vi "624WPI_DashboardReceive DS Packet.vi"(0 "Recv Socket":refnum<k16>, 5 "Log User Data":bool) -> (2 "New Dashboard Data":bool, 3 "Battery":sgl, 4 "Error Strings":string, 6 "Driver Station":T1, 8 "Robot IP Address":string="10.0.0.2", 10 "Status":T3, 12 "Camera IP Address":string="10.0.0.2", 13 "Low Priority User Data":string, 14 "High Priority User Data":string, 15 "Error":T2)   [LabVIEW 2013]
uses:
  <vilib>/Rock Robotics/WPI/Dashboard/WPI_DashboardDStoPCPacketTypeDef.ctl
  <vilib>/Rock Robotics/WPI/Dashboard/WPI_DashboardLogging Global.vi
panel:
  out "Team ID":u16
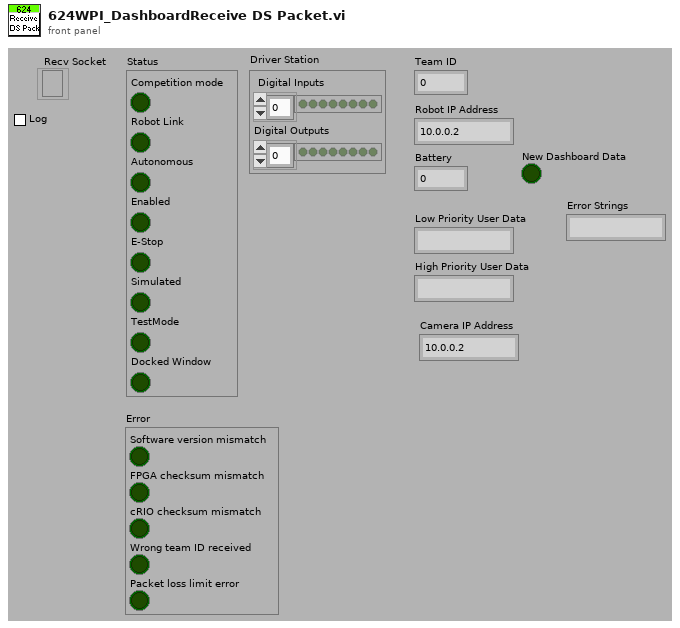
[diagram p1: front panel]
types:
  T1 = cluster{"Digital Inputs":bool[], "Digital Outputs":bool[]}
  T2 = cluster{"Software version mismatch":bool, "FPGA checksum mismatch":bool, "cRIO checksum mismatch":bool, "Wrong team ID received":bool, "Packet loss limit error":bool}
  T3 = cluster{"Competition mode":bool, "Robot Link":bool, "Autonomous":bool, "Enabled":bool, "E-Stop":bool, "Simulated":bool, "TestMode":bool, "Docked Window":bool}
  T4 = typedef "WPI_DashboardDStoPCPacketTypeDef.ctl" = cluster{"Packet Index":u16, "Digital Inputs":u8, "Digital Out":u8, "Battery":u16, "Status":u8, "Error":u8, "Team ID":u16, "VersionMonth1":u8, "VersionMonth2":u8, "VersionDay1":u8, "VersionDay2":u8, "VersionYear1":u8, "VersionYear2":u8, "Revision1":u8, "Revision2":u8, "Robot IP":u32, "UnusedBuffer 2":u8, "ExtraModeFlags":u8, "Reply Packet #":u16}
  T5 = cluster{u16, "Error":cluster{"Software version mismatch":bool, "FPGA checksum mismatch":bool, "cRIO checksum mismatch":bool, "Wrong team ID received":bool, "Packet loss limit error":bool}, "Status":cluster{"Competition mode":bool, "Robot Link":bool, "Autonomous":bool, "Enabled":bool, "E-Stop":bool, "Simulated":bool, "TestMode":bool, "Docked Window":bool}, "Simulator":bool, cluster{"DS Dig Inputs":bool[], "DS Dig Outputs":bool[]}, "Battery":sgl, "name":string}
  T6 = cluster{"DS Dig Inputs":bool[], "DS Dig Outputs":bool[]}
  T7 = typedef "Vector4.ctl" = cluster{"x":sgl, "y":sgl, "z":sgl, "w":sgl}
  T8 = typedef "SkeletonTrackState.ctl" = enum32{"NotTracked", "PositionOnly", "Tracked"}
  T9 = typedef "WPI_JoystickDeviceDataRaw.ctl" = cluster{"axis 1":i8, "axis 2":i8, "axis 3":i8, "axis 4":i8, "axis 5":i8, "axis 6":i8, "Buttons":u16}
  T10 = cluster{"size":u8, "tag":u8, "Version":cluster{"unsigned byte array[0]":u8, "unsigned byte array[1]":u8, "unsigned byte array[2]":u8, "unsigned byte array[3]":u8, "unsigned byte array[4]":u8, "unsigned byte array[5]":u8, "unsigned byte array[6]":u8, "unsigned byte array[7]":u8, "unsigned byte array[8]":u8, "unsigned byte array[9]":u8, "unsigned byte array[10]":u8}, "numPlayers":i8, "flags":u32, "floorClipPlane":T7, "Gravity Normal":cluster{"x":sgl, "y":sgl, "z":sgl}, "size":u8, "tag":u8, "Extra Data":cluster{"TrackingState":cluster{"TrackingState[0]":u8, "TrackingState[1]":u8, "TrackingState[2]":u8, "TrackingState[3]":u8, "TrackingState[4]":u8, "TrackingState[5]":u8, "TrackingState[6]":u8, "TrackingState[7]":u8, "TrackingState[8]":u8, "TrackingState[9]":u8, "TrackingState[10]":u8, "TrackingState[11]":u8, "TrackingState[12]":u8, "TrackingState[13]":u8, "TrackingState[14]":u8, "TrackingState[15]":u8, "TrackingState[16]":u8, "TrackingState[17]":u8, "TrackingState[18]":u8, "TrackingState[19]":u8}, "Position":cluster{"x":sgl, "y":sgl, "z":sgl}, "Quality":u32, "TrackState":T8}, "size":u8, "tag":u8, "Vertices":cluster{"Vertices[0]":cluster{"x":sgl, "y":sgl, "z":sgl}, "Vertices[1]":cluster{"x":sgl, "y":sgl, "z":sgl}, "Vertices[2]":cluster{"x":sgl, "y":sgl, "z":sgl}, "Vertices[3]":cluster{"x":sgl, "y":sgl, "z":sgl}, "Vertices[4]":cluster{"x":sgl, "y":sgl, "z":sgl}, "Vertices[5]":cluster{"x":sgl, "y":sgl, "z":sgl}, "Vertices[6]":cluster{"x":sgl, "y":sgl, "z":sgl}, "Vertices[7]":cluster{"x":sgl, "y":sgl, "z":sgl}, "Vertices[8]":cluster{"x":sgl, "y":sgl, "z":sgl}, "Vertices[9]":cluster{"x":sgl, "y":sgl, "z":sgl}, "Vertices[10]":cluster{"x":sgl, "y":sgl, "z":sgl}, "Vertices[11]":cluster{"x":sgl, "y":sgl, "z":sgl}, "Vertices[12]":cluster{"x":sgl, "y":sgl, "z":sgl}, "Vertices[13]":cluster{"x":sgl, "y":sgl, "z":sgl}, "Vertices[14]":cluster{"x":sgl, "y":sgl, "z":sgl}, "Vertices[15]":cluster{"x":sgl, "y":sgl, "z":sgl}, "Vertices[16]":cluster{"x":sgl, "y":sgl, "z":sgl}, "Vertices[17]":cluster{"x":sgl, "y":sgl, "z":sgl}, "Vertices[18]":cluster{"x":sgl, "y":sgl, "z":sgl}, "Vertices[19]":cluster{"x":sgl, "y":sgl, "z":sgl}}, "size":u8, "tag":u8, "Joystick":T9, "Joystick 2":T9, "size":u8, "tag":u8, "Custom Data":string}[]
  T11 = cluster{"Team ID":u16, "Error":cluster{"Software version mismatch":bool, "FPGA checksum mismatch":bool, "cRIO checksum mismatch":bool, "Wrong team ID received":bool, "Packet loss limit error":bool}, "Status":cluster{"Competition mode":bool, "Robot Link":bool, "Autonomous":bool, "Enabled":bool, "E-Stop":bool, "Simulated":bool, "TestMode":bool, "Docked Window":bool}, "Robot IP":string, "Camera IP":string}
  T12 = cluster{cluster{"Packet #":u8, "High Priority":string, "Error Strings":string, "Low Priority":string}, cluster{"DS Digital In":bool[], "DS Digital Out":bool[]}, "Battery":sgl}
  T13 = cluster{"Packet #":u8, "High Priority":string, "Error Strings":string, "Low Priority":string}
  T14 = cluster{"DS Digital In":bool[], "DS Digital Out":bool[]}
  T15 = cluster{"Team ID":u16, "Error":cluster{"Software version mismatch":bool, "FPGA checksum mismatch":bool, "cRIO checksum mismatch":bool, "Wrong team ID received":bool, "Packet loss limit error":bool}, "Status":cluster{"Competition mode":bool, "Robot Link":bool, "Autonomous":bool, "Enabled":bool, "E-Stop":bool, "Simulated":bool, "TestMode":bool, "Docked Window":bool}, "Camera IP":string, "Camera IP":string}
  T16 = typedef "Protocol Operations.ctl" = enum16{"Unknown", "Keep Alive", "Hello", "Version not supported", "Hello Complete", "Assign", "Update", "No Op"}
  T17 = typedef "Field Data.ctl" = cluster{"Dbl":dbl, "String":string, "Type":T18, "Boolean":bool, "Sequence #":T19}
  T18 = typedef "Field Type.ctl" = enum8{"Invalid", "Bool", "Numeric", "String", "Boolean Array", "Numeric Array", "String Array"}
  T19 = typedef "Sequence.ctl" = u16
  T20 = cluster{"Operation":T16, "Name":string, "Field Value":T17}[]
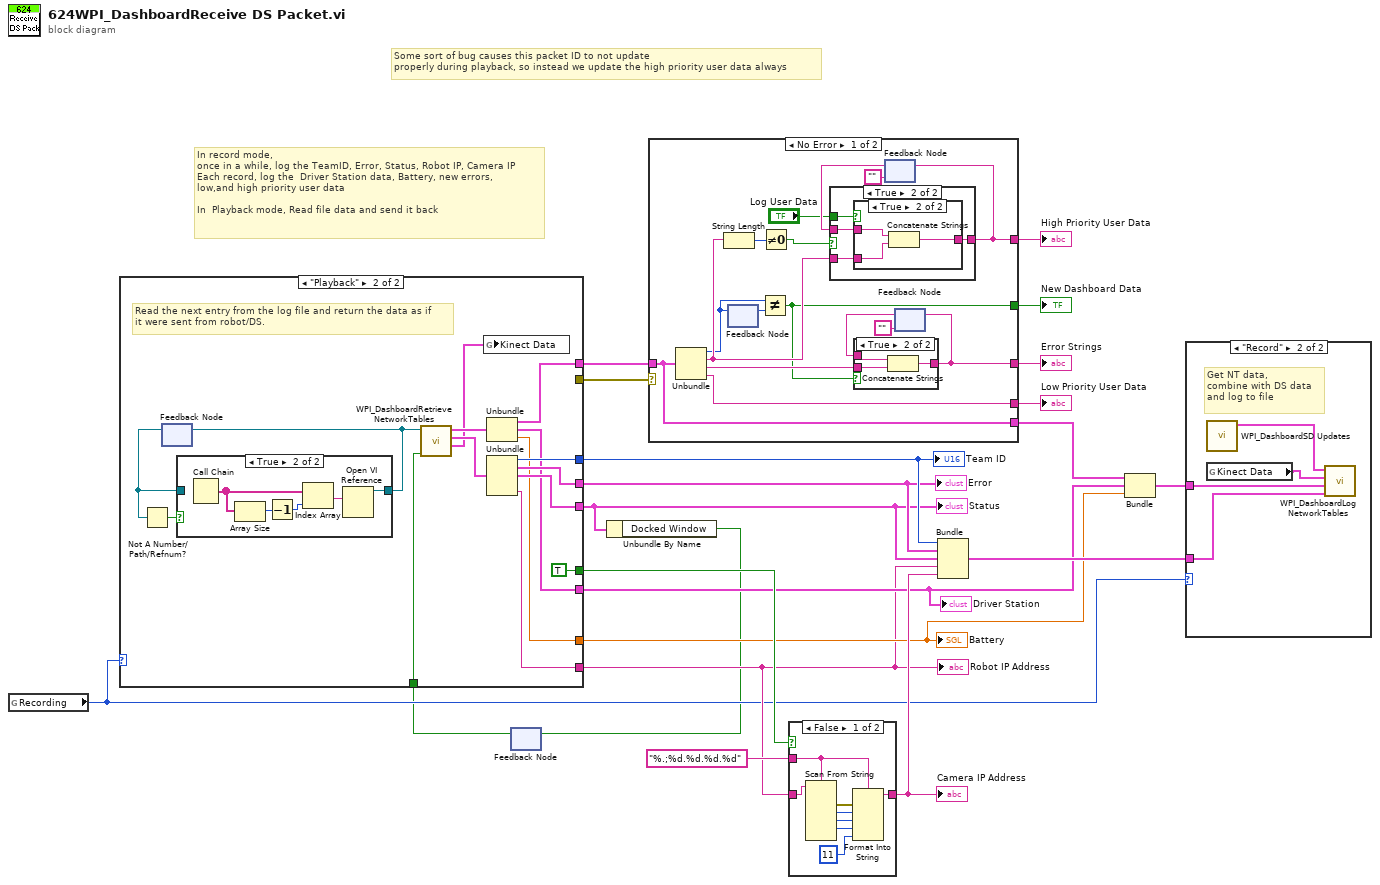
[diagram p0: block diagram]
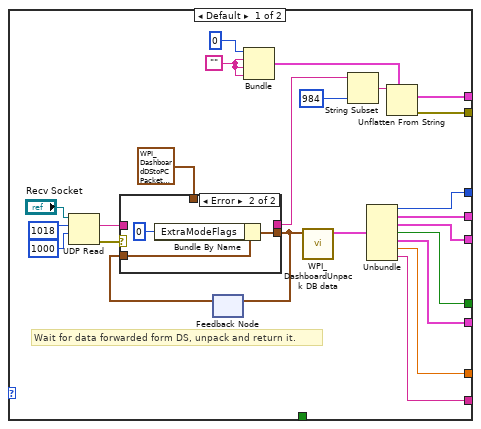
[diagram p3: hidden frame]
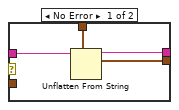
[diagram p4: hidden frame]
diagram:
  # "Some sort of bug causes this packet ID to not update\nproperly during playback, so instead we update the high priority user data always"
  # "In record mode,\nonce in a while, log the TeamID, Error, Status, Robot IP, Camera IP\nEach record, log the  Driver Station data, Battery, new errors,\nlow,and high priority user data\n\nIn  Playback mode, Read file data and send it back"
  n1 = global read "WPI_DashboardLogging Global.vi" "Recording"() -> (w4:enum32{"Stop", "Record", "Playback"})
  n2 = feedback #1() -> (w1:bool)  [unwired: 1 in]
  n3 = case shown="\"Playback\"" w4 {
    tunnel: [w32 _] -> w12
    tunnel: [w31 w66] -> w11
    tunnel: [w29 w64] -> w10
    tunnel: [w28 w63] -> w9
    tunnel: [w27 w62] -> w3
    tunnel: [w26 TRUE] -> w8
    tunnel: [w25 w61] -> w7
    tunnel: [w24 w60] -> w6
    tunnel: [w23 w53] -> w5
    tunnel: w1 -> [_ w55]
    frame Default {
      w39 = ""
      # "Wait for data forwarded form DS, unpack and return it."
      n4 = UDP Read(connection ID="Recv Socket", max size (548)=1018 ("bytes to read"), timeout ms (25000)=1000) -> (data out=w34:string, error out=w33:errorcluster)  [unwired: 1 in, 3 out]
      n5 = feedback #2() -> (w40:T4)  [unwired: 1 in]
      n6 = case shown="Error" w33 {
        tunnel: w34 -> [w49 _]
        tunnel: w40 -> [_ w51]
        tunnel: [w48 w52] -> w22
        tunnel: T4 {"Packet Index"=0, "Digital Inputs"=0, "Digital Out"=0, "Battery"=0, "Status"=0, "Error"=0, "Team ID"=0, "VersionMonth1"=0, "VersionMonth2"=0, "VersionDay1"=0, "VersionDay2"=0, "VersionYear1"=0, "VersionYear2"=0, "Revision1"=0, "Revision2"=0, "Robot IP"=0, "UnusedBuffer 2"=0, "ExtraModeFlags"=0, "Reply Packet #"=0} ("Cluster") -> [w47 _]
        tunnel: [w46 _] -> w42
        frame No Error {
          n7 = Unflatten From String(type=w47, binary string=w49) -> (rest of the binary string=w46:string, value=w48:T4)  [unwired: 1 in, 3 out]
        }
        frame Error {
          n8 = Bundle By Name(cluster=w51, "ExtraModeFlags"=u8 0) -> (w52:T4)
        }
      }
      n9 = feedback-in #2(w22) -> ()
      n10 = Bundle(u8 0, w39, w39, w39) -> (w37:cluster{u8, string, string, string})  [unwired: 1 out]
      n11 = call <vilib>:"WPI_DashboardUnpack DB data.vi"("DB Packed Data"=w22) -> ("output values"=w30:T5)  [unwired: 10 in]
      n12 = String Subset(string=w42, length (rest)=984 ("length (rest)")) -> (substring=w36:string)  [unwired: 1 out]
      n13 = Unbundle(w30) -> (w29:u16, "Error"=w28:T2, "Status"=w27:T3, "Simulator"=w26:bool, w25:T6, "Battery"=w24:sgl, "name"=w23:string)
      n14 = Unflatten From String(type=w37, binary string=w36) -> (value=w31:cluster{u8, string, string, string}, error out=w32:errorcluster)  [unwired: 1 in, 3 out]
    }
    frame "Playback" {
      # "Read the next entry from the log file and return the data as if\nit were sent from robot/DS."
      n15 = feedback #3() -> (w57:refnum<vi>)  [unwired: 1 in]
      n16 = Not A Number/Path/Refnum?(number/path/refnum=w57) -> (NaN/Path/Refnum?=w58:bool)
      n17 = case shown="True" w58 {
        tunnel: w57 -> [w68 _]
        tunnel: [w68 w72] -> w56
        frame False {
        }
        frame True {
          n18 = Call Chain() -> (call chain=w71:string[])
          n19 = Array Size(array=w71) -> (size(s)=w70:i32)
          n20 = Decrement(x=w70) -> (x-1=w69:i32)
          n21 = Index Array(array=w71, index=w69) -> (element=w73:string)
          n22 = Open VI Reference(vi path=w73) -> (vi reference=w72:refnum<vi>)  [unwired: 5 in, 1 out]
        }
      }
      n23 = feedback-in #3(w56) -> ()
      n24 = call <vilib>:"WPI_DashboardRetrieve NetworkTables.vi"("Docked Window"=w55, "VI Refnum"=w56) -> ("Kinect Data"=w54:T10, "Occasional DB Data"=w65:T11, "Frequent DB Data"=w67:T12)  [unwired: 7 in]
      n25 = global write "WPI_DashboardLogging Global.vi" "Kinect Data"(w54) -> ()
      n26 = Unbundle(w67) -> (w66:T13, w61:T14, "Battery"=w60:sgl)
      n27 = Unbundle(w65) -> ("Team ID"=w64:u16, "Error"=w63:T2, "Status"=w62:T3, "Camera IP"=w53:string)  [unwired: 1 out]
    }
  }
  "Battery" <- w6
  "Status" <- w3
  "Error" <- w9
  "Team ID" <- w10
  "Robot IP Address" <- w5
  "Driver Station" <- w7
  n28 = Unbundle By Name(w3) -> ("Docked Window"=w2:bool)
  n29 = feedback-in #1(w2) -> ()
  n30 = case shown="No Error" w12 {
    tunnel: w11 -> [w75 _]
    tunnel: [w79 _] -> w20
    tunnel: [w78 _] -> w19
    tunnel: [w77 _] -> w18
    tunnel: [w76 _] -> w16
    tunnel: [w75 _] -> w15
    frame No Error {
      n31 = Unbundle(w75) -> ("Packet #"=w81:u8, "High Priority"=w82:string, "Error Strings"=w86:string, "Low Priority"=w76:string)
      n32 = String Length(string=w82) -> (length=w83:i32)
      n33 = feedback-in #4(w81) -> ()
      n34 = feedback #4() -> (w80:u8)  [unwired: 1 out]
      n35 = Not Equal?(x=w81, y=w80) -> (x != y?=w77:bool)
      n36 = Not Equal To 0?(x=w83) -> (x != 0?=w74:bool)
      n37 = feedback #5("") -> (w87:string)
      n38 = case shown="True" w74 {
        tunnel: w82 -> [_ w98]
        tunnel: [w94 w97] -> w79
        tunnel: w87 -> [w94 w96]
        tunnel: "Log User Data" -> [_ w95]
        frame False {
        }
        frame True {
          n39 = case shown="True" w95 {
            tunnel: w98 -> [w99 w102]
            tunnel: [w99 w101] -> w97
            tunnel: w96 -> [_ w100]
            frame False {
            }
            frame True {
              n40 = Concatenate Strings(w100, w102) -> (w101:string)
            }
          }
        }
      }
      n41 = feedback-in #5(w79) -> ()
      n42 = feedback #6("") -> (w89:string)
      n43 = case shown="True" w77 {
        tunnel: [w90 w93] -> w78
        tunnel: w89 -> [w90 w92]
        tunnel: w86 -> [_ w91]
        frame False {
        }
        frame True {
          n44 = Concatenate Strings(w92, w91) -> (w93:string)
        }
      }
      n45 = feedback-in #6(w78) -> ()
    }
    frame Error {
    }
  }
  "High Priority User Data" <- w20
  "Error Strings" <- w19
  "New Dashboard Data" <- w18
  "Low Priority User Data" <- w16
  n46 = case shown="False" w8 {
    tunnel: [w105 w111] -> w17
    tunnel: w5 -> [w104 w111]
    tunnel: "%.;%d.%d.%d.%d" ("format string") -> [w103 _]
    frame False {
      n47 = Scan From String(format string=w103, input string=w104) -> (error out=w107:errorcluster, output 1=w108:i32, output 2=w109:i32, output 3=w110:i32)  [unwired: 2 in, 7 out]
      n48 = Format Into String(format string=w103, error in=w107, w108, w109, w110, 11 ("IP Suffix:")) -> (resulting string=w105:string)  [unwired: 1 in, 1 out]
    }
    frame True {
    }
  }
  "Camera IP Address" <- w17
  n49 = Bundle("Team ID"=w10, "Error"=w9, "Status"=w3, "Camera IP"=w5, "Camera IP"=w17) -> (w13:T15)  [unwired: 1 in]
  n50 = Bundle(w15, w7, "Battery"=w6) -> (w14:T12)  [unwired: 1 in]
  n51 = case shown="\"Record\"" w4 {
    tunnel: w14 -> [_ w115]
    tunnel: w13 -> [_ w114]
    frame "Stop", Default {
    }
    frame "Record" {
      # "Get NT data,\ncombine with DS data\nand log to file"
      n52 = call <vilib>:"WPI_DashboardSD Updates.vi"() -> ("Collected Data"=w113:T20)  [unwired: 11 in]
      n53 = global read "WPI_DashboardLogging Global.vi" "Kinect Data"() -> (w112:T10)
      n54 = call <vilib>:"WPI_DashboardLog NetworkTables.vi"("Occasional DB Data"=w114, "Frequent DB Data"=w115, "Kinect Data"=w112, "NT Data Values"=w113) -> ()  [unwired: 8 in]
    }
  }
